vi "Initialize Plugin Settings.vi"(7 "Plugin Engine Settings in":T2, 8 "error in":errorcluster, 11 "Compiled Settings":variant) -> (0 "error out":errorcluster, 3 "Channel Refs":T1, 5 "Plugin Engine Settings out":T2)   [LabVIEW 2026, in "Template Plugin.lvlib" / "Template.lvclass"]
uses:
  Template.lvclass
  Template.lvclass/Template.ctl
  Shared/PluginSettings.ctl
  Shared/GroupedChannelRefs.ctl
  Shared/GroupSettings.ctl
  Shared/ChannelGroups.ctl
  Shared/Compiled.Settings.ctl
  Types/TargetSettings.ctl
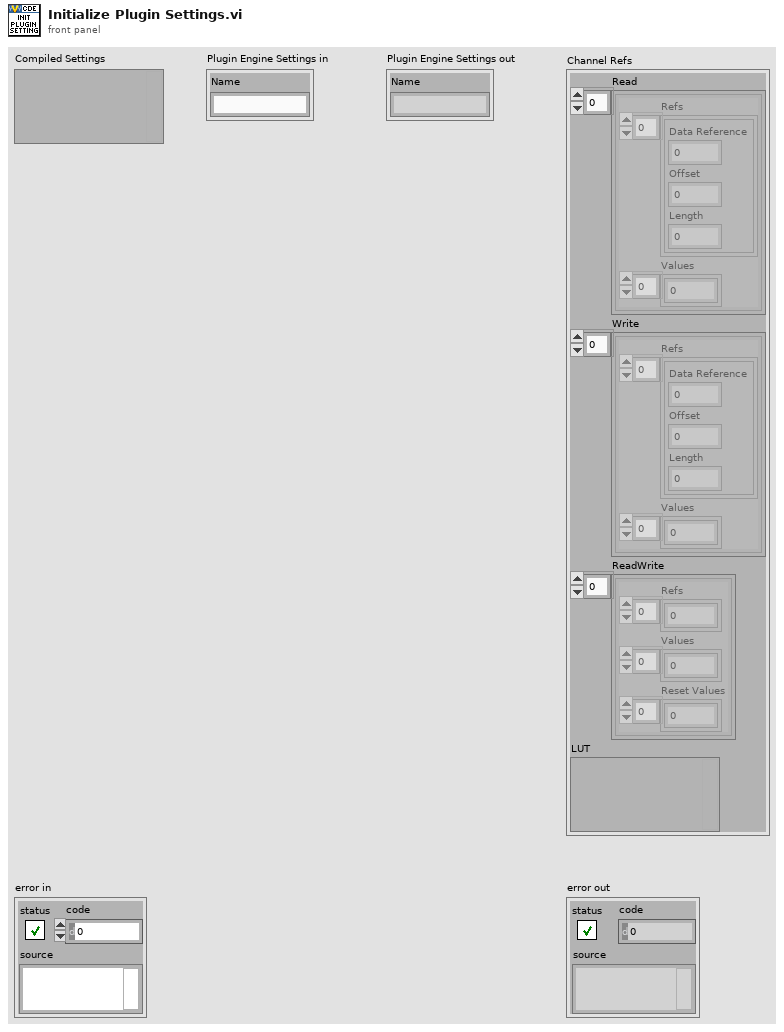
[diagram p1: front panel]
types:
  T1 = cluster{"Read":cluster{"Refs":cluster{"Data Reference":i32, "Offset":u64, "Length":u64}[], "Values":dbl[]}[], "Write":cluster{"Refs":cluster{"Data Reference":i32, "Offset":u64, "Length":u64}[], "Values":dbl[]}[], "ReadWrite":cluster{"Refs":i32[], "Values":dbl[], "Reset Values":dbl[]}[], "LUT":variant}
  T2 = typedef "Template Plugin.lvlib/Template.lvclass/TargetSettings.ctl" = cluster{"Name":string}
  T3 = enum16{"Output/Write", "Input/Read", "Input/ReadWrite"}
  T4 = typedef "Compiled.Settings.ctl" = cluster{"ExampleCustomDevice":T5, "Channel Groups":T6}
  T5 = typedef "PluginSettings.ctl" = cluster{"Name":string, "Properties":cluster{"Low frequency":string, "Low frequency (Hz)":bool[], "High frequency [Hz]":bool, "Frequency : Low Level frequency":dbl[], "Frequency.High frequency":dbl, "I16_PropertyExample":i16, "I16ArrayPropertyExample":i16[], "I32PropertyExample":i32, "I32ArrayPropertyExample":i32[], "I64PropertyExample":i64, "I64ArrayPropertyExample":i64[], "StringArrayPropertyExample":string[], "StringPropertyExample":string, "U16PropertyExample":u16, "U16ArrayPropertyExample":u16[], "U32PropertyExample":u32, "U32ArrayPropertyExample":u32[], "U64PropertyExample":u64, "U64ArrayPropertyExample":u64[], "DependentFilePropertyExample":cluster{"Version":string, "Type":string, "ForceDownload":bool, "RTDestination":string, "SupportedTarget":string, "MD5":string, "Path":string}, "VariantPropertyExample":variant, "TargetOS":string, "TargetRate":dbl}, "Channels":cluster{"TimeChannel":cluster{"Name":string, "Properties":cluster{"Low frequency":string, "Low frequency (Hz)":bool[], "High frequency [Hz]":bool, "Frequency : Low Level frequency":dbl[], "Frequency.High frequency":dbl, "I16PropertyExample":i16, "I16ArrayPropertyExample":i16[], "I32PropertyExample":i32, "I32ArrayPropertyExample":i32[], "I64PropertyExample":i64, "I64ArrayPropertyExample":i64[], "StringArrayPropertyExample":string[], "StringPropertyExample":string, "U16PropertyExample":u16, "U16ArrayPropertyExample":u16[], "U32PropertyExample":u32, "U32ArrayPropertyExample":u32[], "U64PropertyExample":u64, "U64ArrayPropertyExample":u64[], "DependentFilePropertyExample":cluster{"Version":string, "Type":string, "ForceDownload":bool, "RTDestination":string, "SupportedTarget":string, "MD5":string, "Path":string}, "VariantPropertyExample":variant}, "DefaultValue":dbl, "Units":string, "GroupName":string, "Type":string, "Faultable":bool, "Scalable":bool, "ChannelDataReference":i32}[], "FrequencyChannel":cluster{"Name":string, "Properties":cluster{"BinaryStringPropertyExample":string, "BooleanArrayPropertyExample":bool[], "BooleanPropertyExample":bool, "DoubleArrayPropertyExample":dbl[], "DoublePropertyExample":dbl, "I16PropertyExample":i16, "I16ArrayPropertyExample":i16[], "I32PropertyExample":i32, "I32ArrayPropertyExample":i32[], "I64PropertyExample":i64, "I64ArrayPropertyExample":i64[], "StringArrayPropertyExample":string[], "StringPropertyExample":string, "U16PropertyExample":u16, "U16ArrayPropertyExample":u16[], "U32PropertyExample":u32, "U32ArrayPropertyExample":u32[], "U64PropertyExample":u64, "U64ArrayPropertyExample":u64[], "DependentFilePropertyExample":cluster{"Version":string, "Type":string, "ForceDownload":bool, "RTDestination":string, "SupportedTarget":string, "MD5":string, "Path":string}, "VariantPropertyExample":variant}, "DefaultValue":dbl, "Units":string, "GroupName":string, "Type":string, "Faultable":bool, "Scalable":bool, "ChannelDataReference":i32}[]}, "Waveforms":cluster{"AnalogInput":cluster{"Name":string, "Properties":cluster{"Low frequency":string, "Low frequency (Hz)":bool[], "High frequency [Hz]":bool, "Frequency : Low Level frequency":dbl[], "Frequency.High frequency":dbl, "I16PropertyExample":i16, "I16ArrayPropertyExample":i16[], "I32PropertyExample":i32, "I32ArrayPropertyExample":i32[], "I64PropertyExample":i64, "I64ArrayPropertyExample":i64[], "StringArrayPropertyExample":string[], "StringPropertyExample":string, "U16PropertyExample":u16, "U16ArrayPropertyExample":u16[], "U32PropertyExample":u32, "U32ArrayPropertyExample":u32[], "U64PropertyExample":u64, "U64ArrayPropertyExample":u64[], "DependentFilePropertyExample":cluster{"Version":string, "Type":string, "ForceDownload":bool, "RTDestination":string, "SupportedTarget":string, "MD5":string, "Path":string}, "VariantPropertyExample":variant}, "DataType":string, "Units":string, "WaveformDataReference":i32}[]}, "Sections":cluster{"SectionA0":cluster{"Name":string, "Properties":cluster{"BinaryStringPropertyExample":string, "BooleanArrayPropertyExample":bool[], "BooleanPropertyExample":bool, "DoubleArrayPropertyExample":dbl[], "DoublePropertyExample":dbl, "I16PropertyExample":i16, "I16ArrayPropertyExample":i16[], "I32PropertyExample":i32, "I32ArrayPropertyExample":i32[], "I64PropertyExample":i64, "I64ArrayPropertyExample":i64[], "StringArrayPropertyExample":string[], "StringPropertyExample":string, "U16PropertyExample":u16, "U16ArrayPropertyExample":u16[], "U32PropertyExample":u32, "U32ArrayPropertyExample":u32[], "U64PropertyExample":u64, "U64ArrayPropertyExample":u64[], "DependentFilePropertyExample":cluster{"Version":string, "Type":string, "ForceDownload":bool, "RTDestination":string, "SupportedTarget":string, "MD5":string, "Path":string}, "VariantPropertyExample":variant}, "Channels":cluster{"TimeChannel":cluster{"Name":string, "Properties":cluster{"Low frequency":string, "Low frequency (Hz)":bool[], "High frequency [Hz]":bool, "Frequency : Low Level frequency":dbl[], "Frequency.High frequency":dbl, "I16PropertyExample":i16, "I16ArrayPropertyExample":i16[], "I32PropertyExample":i32, "I32ArrayPropertyExample":i32[], "I64PropertyExample":i64, "I64ArrayPropertyExample":i64[], "StringArrayPropertyExample":string[], "StringPropertyExample":string, "U16PropertyExample":u16, "U16ArrayPropertyExample":u16[], "U32PropertyExample":u32, "U32ArrayPropertyExample":u32[], "U64PropertyExample":u64, "U64ArrayPropertyExample":u64[], "DependentFilePropertyExample":cluster{"Version":string, "Type":string, "ForceDownload":bool, "RTDestination":string, "SupportedTarget":string, "MD5":string, "Path":string}, "VariantPropertyExample":variant}, "DefaultValue":dbl, "Units":string, "GroupName":string, "Type":string, "Faultable":bool, "Scalable":bool, "ChannelDataReference":i32}[], "FrequencyChannel":cluster{"Name":string, "Properties":cluster{"BinaryStringPropertyExample":string, "BooleanArrayPropertyExample":bool[], "BooleanPropertyExample":bool, "DoubleArrayPropertyExample":dbl[], "DoublePropertyExample":dbl, "I16PropertyExample":i16, "I16ArrayPropertyExample":i16[], "I32PropertyExample":i32, "I32ArrayPropertyExample":i32[], "I64PropertyExample":i64, "I64ArrayPropertyExample":i64[], "StringArrayPropertyExample":string[], "StringPropertyExample":string, "U16PropertyExample":u16, "U16ArrayPropertyExample":u16[], "U32PropertyExample":u32, "U32ArrayPropertyExample":u32[], "U64PropertyExample":u64, "U64ArrayPropertyExample":u64[], "DependentFilePropertyExample":cluster{"Version":string, "Type":string, "ForceDownload":bool, "RTDestination":string, "SupportedTarget":string, "MD5":string, "Path":string}, "VariantPropertyExample":variant}, "DefaultValue":dbl, "Units":string, "GroupName":string, "Type":string, "Faultable":bool, "Scalable":bool, "ChannelDataReference":i32}[]}, "Waveforms":cluster{"AnalogInput":cluster{"Name":string, "Properties":cluster{"Low frequency":string, "Low frequency (Hz)":bool[], "High frequency [Hz]":bool, "Frequency : Low Level frequency":dbl[], "Frequency.High frequency":dbl, "I16PropertyExample":i16, "I16ArrayPropertyExample":i16[], "I32PropertyExample":i32, "I32ArrayPropertyExample":i32[], "I64PropertyExample":i64, "I64ArrayPropertyExample":i64[], "StringArrayPropertyExample":string[], "StringPropertyExample":string, "U16PropertyExample":u16, "U16ArrayPropertyExample":u16[], "U32PropertyExample":u32, "U32ArrayPropertyExample":u32[], "U64PropertyExample":u64, "U64ArrayPropertyExample":u64[], "DependentFilePropertyExample":cluster{"Version":string, "Type":string, "ForceDownload":bool, "RTDestination":string, "SupportedTarget":string, "MD5":string, "Path":string}, "VariantPropertyExample":variant}, "DataType":string, "Units":string, "WaveformDataReference":i32}[]}}[], "SectionR1":cluster{"Name":string, "Properties":cluster{"Low frequency":string, "Low frequency (Hz)":bool[], "High frequency [Hz]":bool, "Frequency : Low Level frequency":dbl[], "Frequency.High frequency":dbl, "I16PropertyExample":i16, "I16ArrayPropertyExample":i16[], "I32PropertyExample":i32, "I32ArrayPropertyExample":i32[], "I64PropertyExample":i64, "I64ArrayPropertyExample":i64[], "StringArrayPropertyExample":string[], "StringPropertyExample":string, "U16PropertyExample":u16, "U16ArrayPropertyExample":u16[], "U32PropertyExample":u32, "U32ArrayPropertyExample":u32[], "U64PropertyExample":u64, "U64ArrayPropertyExample":u64[], "DependentFilePropertyExample":cluster{"Version":string, "Type":string, "ForceDownload":bool, "RTDestination":string, "SupportedTarget":string, "MD5":string, "Path":string}, "VariantPropertyExample":variant}, "Channels":cluster{"TimeChannel":cluster{"Name":string, "Properties":cluster{"Low frequency":string, "Low frequency (Hz)":bool[], "High frequency [Hz]":bool, "Frequency : Low Level frequency":dbl[], "Frequency.High frequency":dbl, "I16PropertyExample":i16, "I16ArrayPropertyExample":i16[], "I32PropertyExample":i32, "I32ArrayPropertyExample":i32[], "I64PropertyExample":i64, "I64ArrayPropertyExample":i64[], "StringArrayPropertyExample":string[], "StringPropertyExample":string, "U16PropertyExample":u16, "U16ArrayPropertyExample":u16[], "U32PropertyExample":u32, "U32ArrayPropertyExample":u32[], "U64PropertyExample":u64, "U64ArrayPropertyExample":u64[], "DependentFilePropertyExample":cluster{"Version":string, "Type":string, "ForceDownload":bool, "RTDestination":string, "SupportedTarget":string, "MD5":string, "Path":string}, "VariantPropertyExample":variant}, "DefaultValue":dbl, "Units":string, "GroupName":string, "Type":string, "Faultable":bool, "Scalable":bool, "ChannelDataReference":i32}[], "FrequencyChannel":cluster{"Name":string, "Properties":cluster{"BinaryStringPropertyExample":string, "BooleanArrayPropertyExample":bool[], "BooleanPropertyExample":bool, "DoubleArrayPropertyExample":dbl[], "DoublePropertyExample":dbl, "I16PropertyExample":i16, "I16ArrayPropertyExample":i16[], "I32PropertyExample":i32, "I32ArrayPropertyExample":i32[], "I64PropertyExample":i64, "I64ArrayPropertyExample":i64[], "StringArrayPropertyExample":string[], "StringPropertyExample":string, "U16PropertyExample":u16, "U16ArrayPropertyExample":u16[], "U32PropertyExample":u32, "U32ArrayPropertyExample":u32[], "U64PropertyExample":u64, "U64ArrayPropertyExample":u64[], "DependentFilePropertyExample":cluster{"Version":string, "Type":string, "ForceDownload":bool, "RTDestination":string, "SupportedTarget":string, "MD5":string, "Path":string}, "VariantPropertyExample":variant}, "DefaultValue":dbl, "Units":string, "GroupName":string, "Type":string, "Faultable":bool, "Scalable":bool, "ChannelDataReference":i32}[]}, "Sections":cluster{"SectionA0":cluster{"Name":string, "Properties":cluster{"BinaryStringPropertyExample":string, "BooleanArrayPropertyExample":bool[], "BooleanPropertyExample":bool, "DoubleArrayPropertyExample":dbl[], "DoublePropertyExample":dbl, "I16PropertyExample":i16, "I16ArrayPropertyExample":i16[], "I32PropertyExample":i32, "I32ArrayPropertyExample":i32[], "I64PropertyExample":i64, "I64ArrayPropertyExample":i64[], "StringArrayPropertyExample":string[], "StringPropertyExample":string, "U16PropertyExample":u16, "U16ArrayPropertyExample":u16[], "U32PropertyExample":u32, "U32ArrayPropertyExample":u32[], "U64PropertyExample":u64, "U64ArrayPropertyExample":u64[], "DependentFilePropertyExample":cluster{"Version":string, "Type":string, "ForceDownload":bool, "RTDestination":string, "SupportedTarget":string, "MD5":string, "Path":string}, "VariantPropertyExample":variant}, "Channels":cluster{"TimeChannel":cluster{"Name":string, "Properties":cluster{"Low frequency":string, "Low frequency (Hz)":bool[], "High frequency [Hz]":bool, "Frequency : Low Level frequency":dbl[], "Frequency.High frequency":dbl, "I16PropertyExample":i16, "I16ArrayPropertyExample":i16[], "I32PropertyExample":i32, "I32ArrayPropertyExample":i32[], "I64PropertyExample":i64, "I64ArrayPropertyExample":i64[], "StringArrayPropertyExample":string[], "StringPropertyExample":string, "U16PropertyExample":u16, "U16ArrayPropertyExample":u16[], "U32PropertyExample":u32, "U32ArrayPropertyExample":u32[], "U64PropertyExample":u64, "U64ArrayPropertyExample":u64[], "DependentFilePropertyExample":cluster{"Version":string, "Type":string, "ForceDownload":bool, "RTDestination":string, "SupportedTarget":string, "MD5":string, "Path":string}, "VariantPropertyExample":variant}, "DefaultValue":dbl, "Units":string, "GroupName":string, "Type":string, "Faultable":bool, "Scalable":bool, "ChannelDataReference":i32}[], "FrequencyChannel":cluster{"Name":string, "Properties":cluster{"BinaryStringPropertyExample":string, "BooleanArrayPropertyExample":bool[], "BooleanPropertyExample":bool, "DoubleArrayPropertyExample":dbl[], "DoublePropertyExample":dbl, "I16PropertyExample":i16, "I16ArrayPropertyExample":i16[], "I32PropertyExample":i32, "I32ArrayPropertyExample":i32[], "I64PropertyExample":i64, "I64ArrayPropertyExample":i64[], "StringArrayPropertyExample":string[], "StringPropertyExample":string, "U16PropertyExample":u16, "U16ArrayPropertyExample":u16[], "U32PropertyExample":u32, "U32ArrayPropertyExample":u32[], "U64PropertyExample":u64, "U64ArrayPropertyExample":u64[], "DependentFilePropertyExample":cluster{"Version":string, "Type":string, "ForceDownload":bool, "RTDestination":string, "SupportedTarget":string, "MD5":string, "Path":string}, "VariantPropertyExample":variant}, "DefaultValue":dbl, "Units":string, "GroupName":string, "Type":string, "Faultable":bool, "Scalable":bool, "ChannelDataReference":i32}[]}, "Waveforms":cluster{"AnalogInput":cluster{"Name":string, "Properties":cluster{"Low frequency":string, "Low frequency (Hz)":bool[], "High frequency [Hz]":bool, "Frequency : Low Level frequency":dbl[], "Frequency.High frequency":dbl, "I16PropertyExample":i16, "I16ArrayPropertyExample":i16[], "I32PropertyExample":i32, "I32ArrayPropertyExample":i32[], "I64PropertyExample":i64, "I64ArrayPropertyExample":i64[], "StringArrayPropertyExample":string[], "StringPropertyExample":string, "U16PropertyExample":u16, "U16ArrayPropertyExample":u16[], "U32PropertyExample":u32, "U32ArrayPropertyExample":u32[], "U64PropertyExample":u64, "U64ArrayPropertyExample":u64[], "DependentFilePropertyExample":cluster{"Version":string, "Type":string, "ForceDownload":bool, "RTDestination":string, "SupportedTarget":string, "MD5":string, "Path":string}, "VariantPropertyExample":variant}, "DataType":string, "Units":string, "WaveformDataReference":i32}[]}}[]}}[]}}
  T6 = typedef "ChannelGroups.ctl" = cluster{"Channel Refs":T7, "Group Settings":T8[]}
  T7 = typedef "GroupedChannelRefs.ctl" = cluster{"Read":cluster{"Refs":cluster{"Data Reference":i32, "Offset":u64, "Length":u64}[], "Values":dbl[]}[], "Write":cluster{"Refs":cluster{"Data Reference":i32, "Offset":u64, "Length":u64}[], "Values":dbl[]}[], "ReadWrite":cluster{"Refs":i32[], "Values":dbl[], "Reset Values":dbl[]}[], "LUT":variant}
  T8 = typedef "GroupSettings.ctl" = cluster{"Name":string, "Type":enum16{"Output/Write", "Input/Read", "Input/ReadWrite"}, "Channel Settings":void[]}
  T9 = cluster{"Name":string, "TypeName":string, "ChannelProperties":variant}[]
  T10 = cluster{"Name":string, "Type":enum16{"Output/Write", "Input/Read", "Input/ReadWrite"}, "Channel Settings":cluster{"Name":string, "TypeName":string, "ChannelProperties":variant}[]}[]
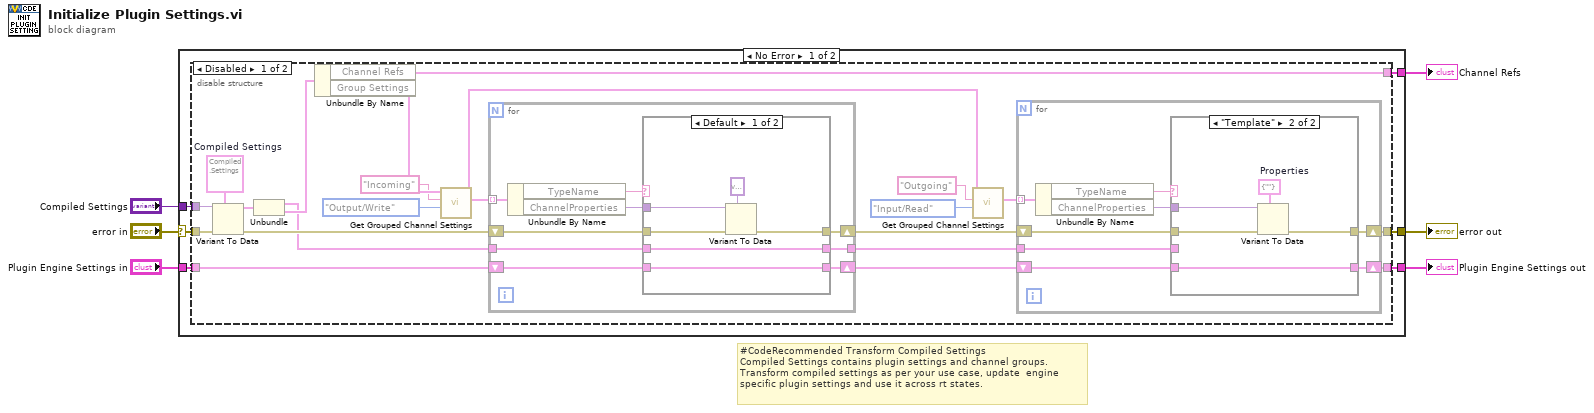
[diagram p0: block diagram]
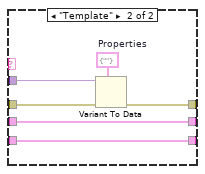
[diagram p2: hidden frame]
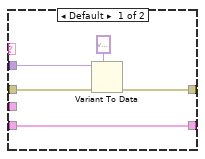
[diagram p3: hidden frame]
diagram:
  # "#CodeRecommended Transform Compiled Settings\nCompiled Settings contains plugin settings and channel groups.\nTransform compiled settings as per your use case, update  engine\nspecific plugin settings and use it across rt states."
  n1 = case shown="No Error" "error in" {
    selector: "error in" -> [w11 w77]
    tunnel: [w12 w77] -> w5
    tunnel: [w7 w76] -> w4
    tunnel: "Plugin Engine Settings in" -> [w8 w76]
    tunnel: "Compiled Settings" -> [w10 _]
    tunnel: [w9 _] -> w1
    frame No Error {
      n2 = disable-structure shown="Disabled" {
        disable-tunnel: [w32 w75] -> w12
        disable-tunnel: w11 -> [w34 w75]
        disable-tunnel: w10 -> [w30 _]
        disable-tunnel: [w17 _] -> w9
        disable-tunnel: w8 -> [w29 w74]
        disable-tunnel: [w13 w74] -> w7
        frame Disabled {
          w28 = T4 {"ExampleCustomDevice"={"Name"="", "Properties"={"Low frequency"="", "Low frequency (Hz)"=[], "High frequency [Hz]"=FALSE, "Frequency : Low Level frequency"=[], "Frequency.High frequency"=0.0, "I16_PropertyExample"=0, "I16ArrayPropertyExample"=[], "I32PropertyExample"=0, "I32ArrayPropertyExample"=[], "I64PropertyExample"=0, "I64ArrayPropertyExample"=[], "StringArrayPropertyExample"=[], "StringPropertyExample"="", "U16PropertyExample"=0, "U16ArrayPropertyExample"=[], "U32PropertyExample"=0, "U32ArrayPropertyExample"=[], "U64PropertyExample"=0, "U64ArrayPropertyExample"=[], "DependentFilePropertyExample"={"Version"="", "Type"="", "ForceDownload"=FALSE, "RTDestination"="", "SupportedTarget"="", "MD5"="", "Path"=""}, "VariantPropertyExample"=variant(cluster{"TimeChannel":cluster{"Name":string, "Properties":cluster{"Low frequency":string, "Low frequency (Hz)":bool[], "High frequency [Hz]":bool, "Frequency : Low Level frequency":dbl[], "Frequency.High frequency":dbl, "I16PropertyExample":i16, "I16ArrayPropertyExample":i16[], "I32PropertyExample":i32, "I32ArrayPropertyExample":i32[], "I64PropertyExample":i64, "I64ArrayPropertyExample":i64[], "StringArrayPropertyExample":string[], "StringPropertyExample":string, "U16PropertyExample":u16, "U16ArrayPropertyExample":u16[], "U32PropertyExample":u32, "U32ArrayPropertyExample":u32[], "U64PropertyExample":u64, "U64ArrayPropertyExample":u64[], "DependentFilePropertyExample":cluster{"Version":string, "Type":string, "ForceDownload":bool, "RTDestination":string, "SupportedTarget":string, "MD5":string, "Path":string}, "VariantPropertyExample":variant}, "DefaultValue":dbl, "Units":string, "GroupName":string, "Type":string, "Faultable":bool, "Scalable":bool, "ChannelDataReference":i32}[], "FrequencyChannel":cluster{"Name":string, "Properties":cluster{"BinaryStringPropertyExample":string, "BooleanArrayPropertyExample":bool[], "BooleanPropertyExample":bool, "DoubleArrayPropertyExample":dbl[], "DoublePropertyExample":dbl, "I16PropertyExample":i16, "I16ArrayPropertyExample":i16[], "I32PropertyExample":i32, "I32ArrayPropertyExample":i32[], "I64PropertyExample":i64, "I64ArrayPropertyExample":i64[], "StringArrayPropertyExample":string[], "StringPropertyExample":string, "U16PropertyExample":u16, "U16ArrayPropertyExample":u16[], "U32PropertyExample":u32, "U32ArrayPropertyExample":u32[], "U64PropertyExample":u64, "U64ArrayPropertyExample":u64[], "DependentFilePropertyExample":cluster{"Version":string, "Type":string, "ForceDownload":bool, "RTDestination":string, "SupportedTarget":string, "MD5":string, "Path":string}, "VariantPropertyExample":variant}, "DefaultValue":dbl, "Units":string, "GroupName":string, "Type":string, "Faultable":bool, "Scalable":bool, "ChannelDataReference":i32}[]} {"TimeChannel"=[], "FrequencyChannel"=[]}), "TargetOS"="", "TargetRate"=0.0}, "Channels"={"TimeChannel"=[], "FrequencyChannel"=[]}, "Waveforms"={"AnalogInput"=[]}, "Sections"={"SectionA0"=[], "SectionR1"=[]}}, "Channel Groups"={"Channel Refs"={"Read"=[], "Write"=[], "ReadWrite"=[], "LUT"=variant}, "Group Settings"=[]}}  # Compiled Settings
          n3 = Variant To Data(error in=w34, type=w28, Variant=w30) -> (data=w27:T4, error out=w33:errorcluster)
          n4 = Unbundle(w27) -> ("ExampleCustomDevice"=w22:T5, "Channel Groups"=w26:T6)
          n5 = Unbundle By Name(w26) -> ("Channel Refs"=w17:T7, "Group Settings"=w25:T8[])
          n6 = call "Get Grouped Channel Settings.vi"("Type"=T3."Output/Write", "Group Name"="Incoming", "Group Settings"=w25) -> ("Channel Settings"=w21:T9, "Group Settings"=w18:T10)  [unwired: 6 in, 1 out]
          n7 = for {
            tunnel: w21 -> [w41] mode=indexing
            tunnel: w22 -> [w38]
            shift-right: [w37] -> w14
            shift-left: w29 -> [w36]
            tunnel: [w35] -> w15
            shift-right: [w42] -> w31
            shift-left: w33 -> [w43]
            n8 = Unbundle By Name(w41) -> ("TypeName"=w40:string, "ChannelProperties"=w39:variant)
            n9 = case "Incoming" shown="Default" w40 {
              tunnel: w39 -> [w45 w51]
              tunnel: w38 -> [w46 w53]
              tunnel: [w47 w52] -> w37
              tunnel: w36 -> [w47 w52]
              tunnel: [w46 w53] -> w35
              tunnel: w43 -> [w49 w55]
              tunnel: [w48 w54] -> w42
              frame Default {
                n10 = Variant To Data(error in=w49, type=variant, Variant=w45) -> (error out=w48:errorcluster)  [unwired: 1 out]
              }
              frame "Template" {
                w50 = cluster{string} {""}  # Properties
                n11 = Variant To Data(error in=w55, type=w50, Variant=w51) -> (error out=w54:errorcluster)  [unwired: 1 out]
              }
            }
          }
          n12 = call "Get Grouped Channel Settings.vi"("Type"=T3."Input/Read", "Group Name"="Outgoing", "Group Settings"=w18) -> ("Channel Settings"=w16:T9)  [unwired: 6 in, 2 out]
          n13 = for {
            tunnel: w16 -> [w61] mode=indexing
            tunnel: w15 -> [w58]
            shift-right: [w57] -> w13
            shift-left: w14 -> [w56]
            shift-right: [w62] -> w32
            shift-left: w31 -> [w63]
            n14 = Unbundle By Name(w61) -> ("TypeName"=w60:string, "ChannelProperties"=w59:variant)
            n15 = case "Outgoing" shown="\"Template\"" w60 {
              tunnel: w59 -> [w65 w70]
              tunnel: w58 -> [_ _]
              tunnel: [w66 w71] -> w57
              tunnel: w56 -> [w66 w71]
              tunnel: w63 -> [w68 w73]
              tunnel: [w67 w72] -> w62
              frame Default {
                n16 = Variant To Data(error in=w68, type=variant, Variant=w65) -> (error out=w67:errorcluster)  [unwired: 1 out]
              }
              frame "Template" {
                w69 = cluster{string} {""}  # Properties
                n17 = Variant To Data(error in=w73, type=w69, Variant=w70) -> (error out=w72:errorcluster)  [unwired: 1 out]
              }
            }
          }
        }
        frame Enabled {
        }
      }
    }
    frame Error {
    }
  }
  "error out" <- w5
  "Plugin Engine Settings out" <- w4
  "Channel Refs" <- w1
